vi "CAN open.vi"(4 "error in (no error)":errorcluster, 5 "Baud rate":i32(ring) items=["1M Baud", "500K Baud", "250K Baud", "125K Baud", "100K Baud", "62K Baud", "50K Baud"], 6 "Channel":u32, 7 "CANopen in":refnum<class "CANopen.lvclass">) -> (0 "error out":errorcluster, 3 "CANopen out":refnum<class "CANopen.lvclass">)   [LabVIEW 2017, in "canopen.lvlib" / "CANopen.lvclass"]
doc: "Establishes a connection with the CAN bus using the given parameters."
uses:
  CANopen.lvclass
  CANopen.lvclass/CANopen.ctl
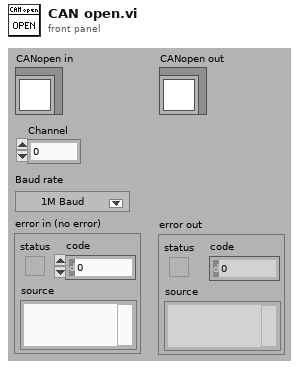
[diagram p1: front panel]
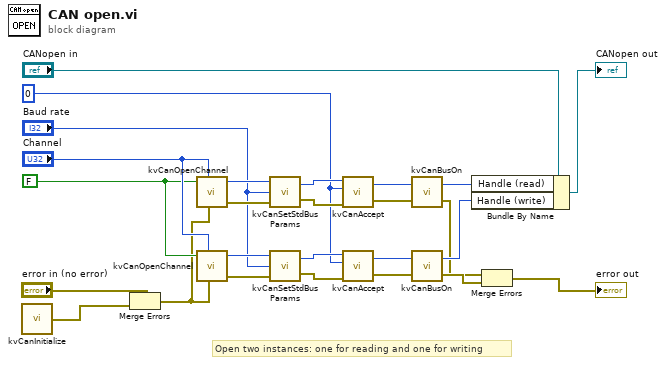
[diagram p0: block diagram]
diagram:
  w4 = FALSE ("WantExclusive")
  w5 = u32 0 ("Envelope Mask or Code")
  # "Open two instances: one for reading and one for writing"
  n1 = call <userlib>:"kvCanInitialize.vi"() -> ("error out (no error)"=w17:errorcluster)
  n2 = Merge Errors("error in (no error)", w17) -> (w1:errorcluster)
  n3 = call <userlib>:"kvCanOpenChannel.vi"("WantExclusive"=w4, "CAN Channel Number"="Channel", "error in (no error)"=w1) -> ("Opened Channel Handle\n(output only)"=w8:i32, "error out"=w9:errorcluster)  [unwired: 2 in]
  n4 = call <userlib>:"kvCanOpenChannel.vi"("WantExclusive"=w4, "CAN Channel Number"="Channel", "error in (no error)"=w1) -> ("Opened Channel Handle\n(output only)"=w26:i32, "error out"=w25:errorcluster)  [unwired: 2 in]
  n5 = call <userlib>:"kvCanSetStdBusParams.vi"("error in (no error)"=w9, "Standard CAN Baud Rate"="Baud rate", "Channel Handle (input only)"=w8) -> ("error out"=w11:errorcluster, "Channel Handle (ouput only)"=w10:i32)
  n6 = call <userlib>:"kvCanSetStdBusParams.vi"("error in (no error)"=w25, "Standard CAN Baud Rate"="Baud rate", "Channel Handle (input only)"=w26) -> ("error out"=w23:errorcluster, "Channel Handle (ouput only)"=w24:i32)
  n7 = call <userlib>:"kvCanAccept.vi"("error in (no error)"=w11, "Envelope Mask or Code"=w5, "Channel Handle (input only)"=w10) -> ("error out"=w13:errorcluster, "Channel Handle (ouput only)"=w12:i32)  [unwired: 1 in]
  n8 = call <userlib>:"kvCanAccept.vi"("error in (no error)"=w23, "Envelope Mask or Code"=w5, "Channel Handle (input only)"=w24) -> ("error out"=w21:errorcluster, "Channel Handle (ouput only)"=w22:i32)  [unwired: 1 in]
  n9 = call <userlib>:"kvCanBusOn.vi"("error in (no error)"=w13, "Channel Handle (input only)"=w12) -> ("error out"=w2:errorcluster, "Channel Handle (ouput only)"=w3:i32)
  n10 = call <userlib>:"kvCanBusOn.vi"("error in (no error)"=w21, "Channel Handle (input only)"=w22) -> ("error out"=w14:errorcluster, "Channel Handle (ouput only)"=w15:i32)
  n11 = Bundle By Name(cluster="CANopen in", "Handle (read)"=w3, "Handle (write)"=w15) -> (→"CANopen out":refnum<class "CANopen.lvclass">)
  n12 = Merge Errors(w2, w14) -> (→"error out":errorcluster)
